vi "Build Grid 14B.vi"(11 "Text":string) -> (1 "Rock Lines":cluster{"Array":u32[][]}[](array[cluster]), 3 "Array":T1[][](array[typedef]), 5 "Start":i32[](array[numeric]))   [LabVIEW 2020]
uses:
  RB ENUM_Space ID.ctl
  5b1ab79e-a290-4079-acbe-56719b58bcf7.vi
  <vilib>/Comparison/Equal/Equal Functor/Equal Functor.lvclass
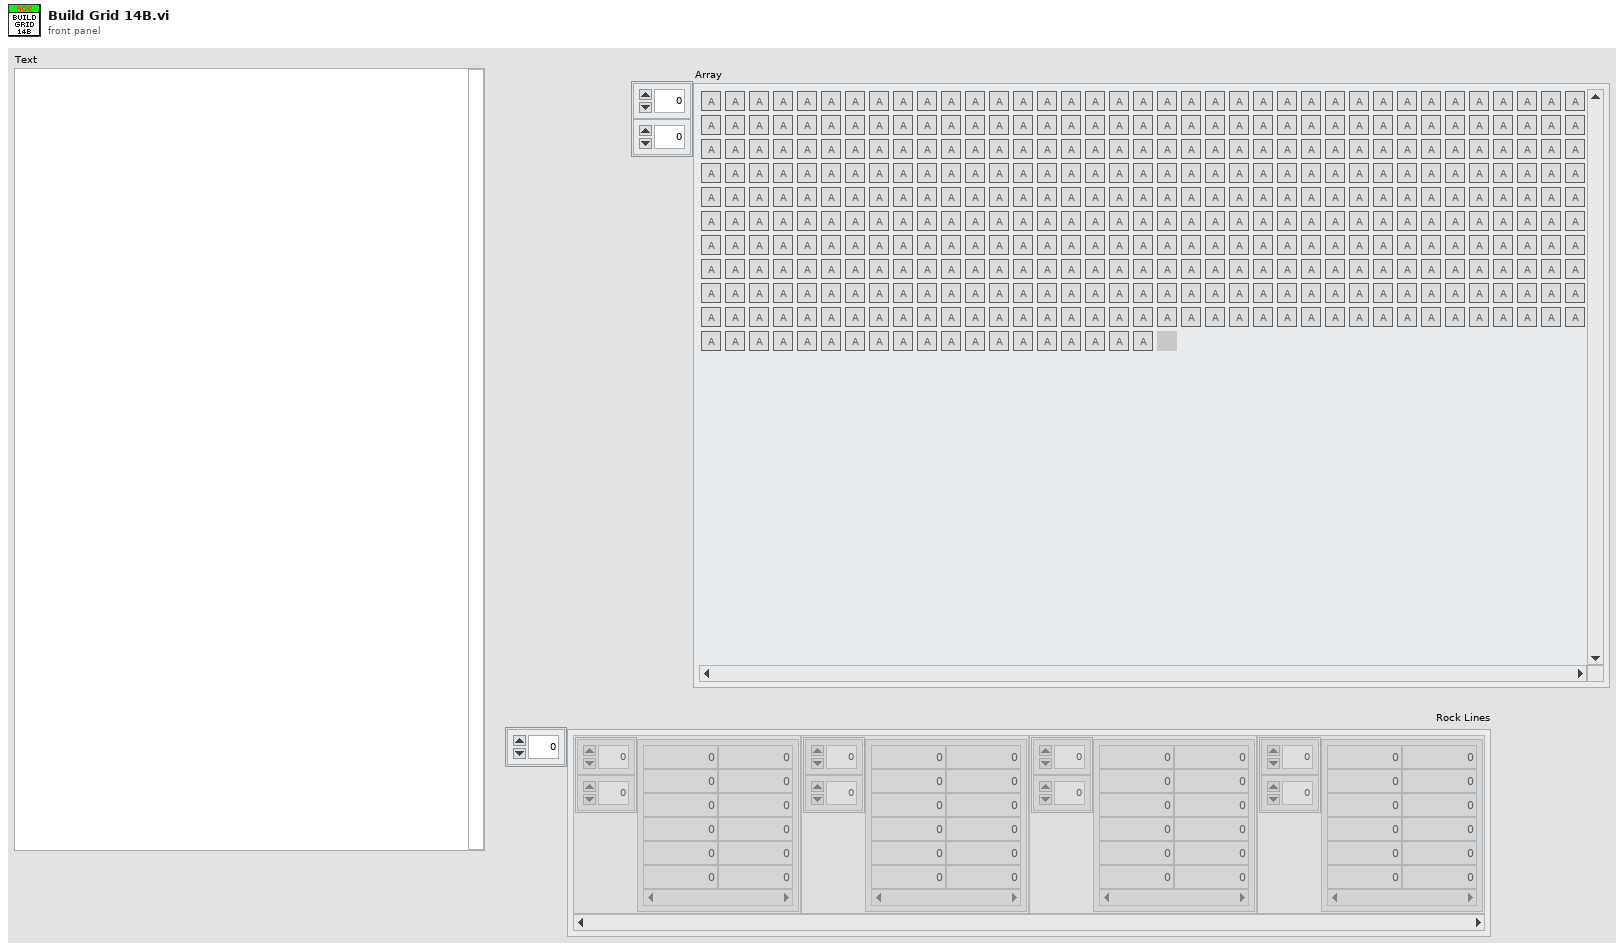
[diagram p1: front panel]
types:
  T1 = typedef "RB ENUM_Space ID.ctl" = enum32{"Air", "Sand", "Rock", "Start", "Abyss"}
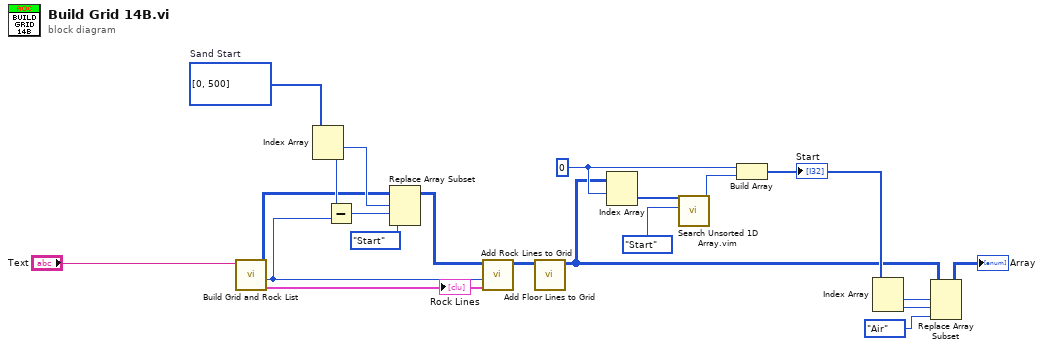
[diagram p0: block diagram]
diagram:
  w8 = 0 ("index (row)")
  w12 = i32[] [0, 500]  # Sand Start
  n1 = call "Build Grid and Rock List.vi"("text data"="Text") -> ("Rock Lines"=w20:cluster{"Array":u32[][]}[], "Column Offset"=w21:i32, "Grig"=w13:T1[][])  [unwired: 8 in]
  "Rock Lines" <- w20
  n2 = Index Array(array=w12) -> (element #1=w16:i32, element #2=w15:i32)  [unwired: 2 in]
  n3 = Subtract(x=w15, y=w21) -> (x-y=w11:i32)
  n4 = Replace Array Subset(array=w13, new element=RB_ENUM_Space_ID."Start" ("Space"), index (row)=w16, index (col)=w11) -> (w17:T1[][])
  n5 = call "Add Rock Lines to Grid.vi"("Rock Lines"=w20, "Column Offset"=w21, "Grig in"=w17) -> ("Grig out"=w18:T1[][])  [unwired: 8 in]
  n6 = call "Add Floor Lines to Grid.vi"("Grig in"=w18) -> ("output array"=w1:T1[][])  [unwired: 10 in]
  n7 = Index Array(array=w1, index (row)=w8) -> (element=w10:T1[])  [unwired: 1 in]
  n8 = call "Search Unsorted 1D Array.vim"("element"=RB_ENUM_Space_ID."Start" ("Space"), "unsorted 1D array"=w10) -> ("index of element"=w9:i32)  [unwired: 9 in]
  n9 = Build Array(w8, w9) -> (w5:i32[])
  "Start" <- w5
  n10 = Index Array(array=w5) -> (element #1=w4:i32, element #2=w3:i32)  [unwired: 2 in]
  n11 = Replace Array Subset(array=w1, new element=RB_ENUM_Space_ID."Air" ("new element/subarray"), index (row)=w4, index (col)=w3) -> (→"Array":T1[][])
